vi "US300 Depth Sensor Driver.vi"() -> ()   [LabVIEW 2011]
panel:
  out "PSI":dbl
  out "Actual Depth 2":dbl
  out "Absolute Depth":dbl
  in  "Atm":dbl
  out "Actual Depth (m)":dbl(slide)
  out "Absolute Depth (m)":dbl(slide)
  in  "Density of Water":dbl
  out "Psi":dbl(graph)
  out "Psi":dbl(knob)
  in  "Wait ms":dbl
  out "error out":errorcluster
  out "Raw Voltage":dbl(graph)
  in  "stop":bool
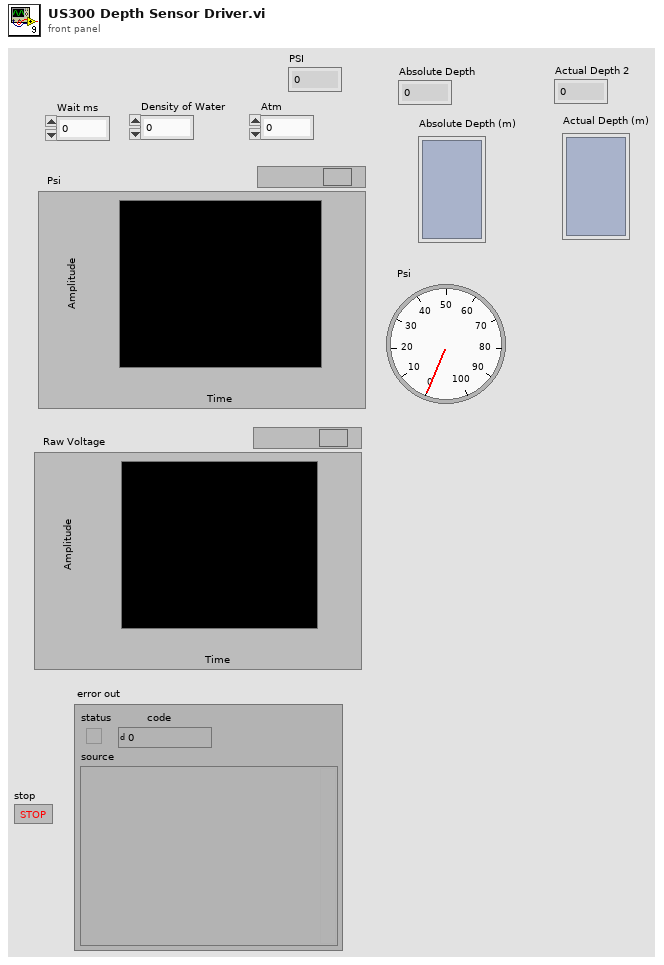
[diagram p1: front panel]
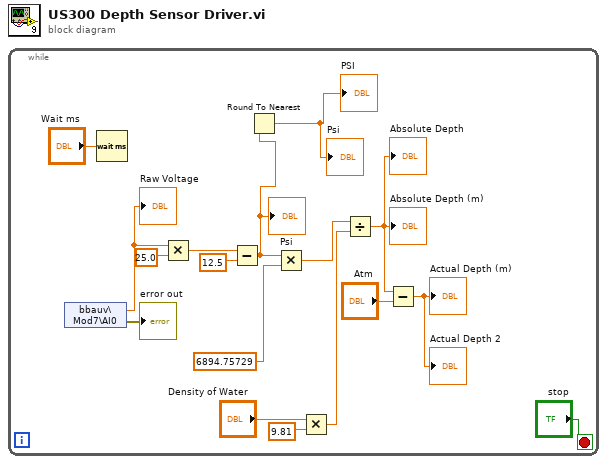
[diagram p0: block diagram]
diagram:
  n1 = while {
    stop <- "stop" stop-if-true
    n2 = shared-variable "bbauv\\Mod7\\AI0"() -> (w14:dbl, error out=→"error out":errorcluster)  [unwired: 1 in]
    "Raw Voltage" <- w14
    n3 = Wait (ms)(milliseconds to wait="Wait ms") -> ()  [unwired: 1 out]
    n4 = Multiply(x=w14, y=25.0) -> (x*y=w12:dbl)
    n5 = Subtract(x=w12, y=12.5) -> (x-y=w2:dbl)
    "Psi" <- w2
    n6 = Round To Nearest(number=w2) -> (nearest integer value=→"Psi" →"PSI":dbl)
    n7 = Multiply(x=w2, y=6894.75729) -> (x*y=w6:dbl)
    n8 = Multiply(x="Density of Water", y=9.81) -> (x*y=w8:dbl)
    n9 = Divide(x=w6, y=w8) -> (x/y=w4:dbl)
    "Absolute Depth (m)" <- w4
    "Absolute Depth" <- w4
    n10 = Subtract(x=w4, y="Atm") -> (x-y=→"Actual Depth (m)" →"Actual Depth 2":dbl)
  }
